vi "Acquire Data.vi"(8 "error in (no error)":errorcluster, 11 "Acquisition in":refnum<class "Acquisition.lvclass">) -> (0 "error out":errorcluster, 3 "Acquisition out":refnum<class "Acquisition.lvclass">)   [LabVIEW 2020]
doc: "Perform the acquisition. Replace the contents of this diagram with calls to acquisition hardware."
uses:
  Acquisition.lvlib
  Workers/Acquisition/Acquisition.lvclass
  C:/Program Files (x86)/National Instruments/LabVIEW 2020/vi.lib/addons/_Workers/Library/Classes/Worker/Worker.lvclass
  C:/Program Files (x86)/National Instruments/LabVIEW 2020/vi.lib/addons/_Workers/Library/Classes/Workers Object/Workers Object.lvclass
  C:/Users/yaoli/Desktop/JKISMPP Continuous Meausrement and Logging/Workers/Acquisition/Acquisition.lvclass
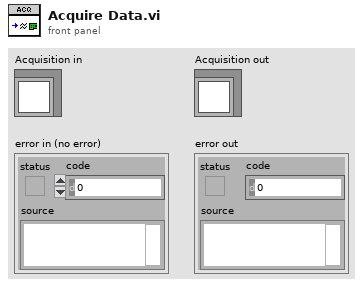
[diagram p1: front panel]
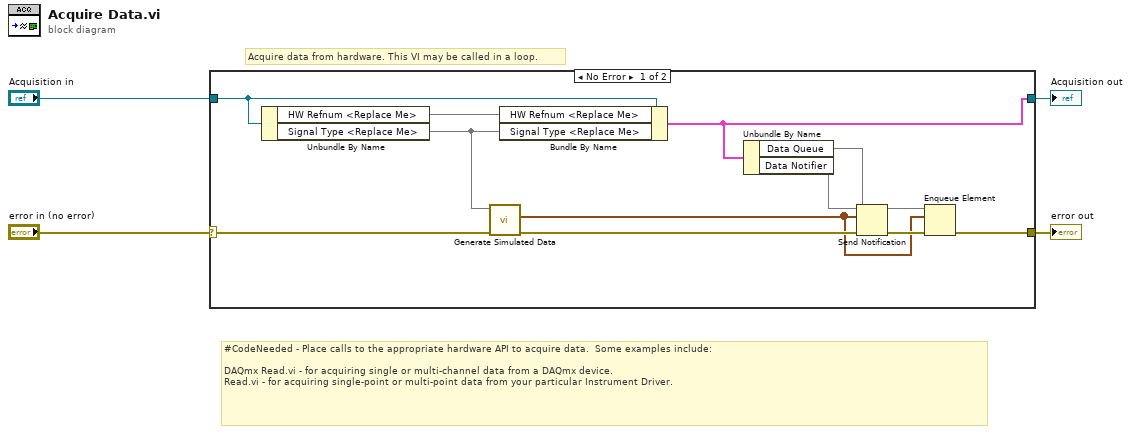
[diagram p0: block diagram]
diagram:
  # "Acquire data from hardware. This VI may be called in a loop."
  # "#CodeNeeded - Place calls to the appropriate hardware API to acquire data.  Some examples include:\n\nDAQmx Read.vi - for acquiring single or multi-channel data from a DAQmx device.\nRead.vi - for acquiring single-point or multi-point data from your particular Instrument Driver."
  n1 = case shown="No Error" "error in (no error)" {
    selector: "error in (no error)" -> [w15 w16]
    tunnel: [w10 w16] -> w3
    tunnel: "Acquisition in" -> [w12 w17]
    tunnel: [w9 w17] -> w1
    frame No Error {
      n2 = Unbundle By Name(w12) -> ("HW Refnum <Replace Me>"=w13, "Signal Type <Replace Me>"=w14)
      n3 = call "Generate Simulated Data.vi"("error in (no error)"=w15, "Signal Type"=w14) -> ("error out"=w11:errorcluster, "Graph Data"=w6:waveform(dbl)[])  [unwired: 8 in]
      n4 = Bundle By Name(cluster=w12, "HW Refnum <Replace Me>"=w13, "Signal Type <Replace Me>"=w14) -> (w9:cluster{})
      n5 = Unbundle By Name(w9) -> ("Data Queue"=w5, "Data Notifier"=w7)
      n6 = Send Notification(notification=w6, notifier=w7, error in (no error)=w11) -> (error out=w8:errorcluster)  [unwired: 1 out]
      n7 = Enqueue Element(queue=w5, element=w6, error in (no error)=w8) -> (error out=w10:errorcluster)  [unwired: 1 in, 2 out]
    }
    frame Error {
    }
  }
  "Acquisition out" <- w1
  "error out" <- w3
